vi "SIAM-DecodeDigitalReturn.vi"(10 "?":i32 format="%.0b", 11 "Array 2":T1(array[cluster])=[{"Digital-out"=enum."cam1", "Boolean"=FALSE}, {"Digital-out"=enum."cam2", "Boolean"=FALSE}, {"Digital-out"=enum."led2", "Boolean"=FALSE}, {"Digital-out"=enum."led3", "Boolean"=FALSE}, {"Digital-out"=enum."led4", "Boolean"=FALSE}, {"Digital-out"=enum."led5", "Boolean"=FALSE}, {"Digital-out"=enum."led5", "Boolean"=FALSE}, {"Digital-out"=enum."led7", "Boolean"=FALSE}, {"Digital-out"=enum."led8", "Boolean"=FALSE}, {"Digital-out"=enum."durchR", "Boolean"=FALSE}, {"Digital-out"=enum."tsm-pwr", "Boolean"=FALSE}, {"Digital-out"=enum."dc-pwr", "Boolean"=FALSE}, {"Digital-out"=enum."laser-pwr", "Boolean"=FALSE}, {"Digital-out"=enum."Laser0", "Boolean"=FALSE}, {"Digital-out"=enum."Laser1", "Boolean"=FALSE}, {"Digital-out"=enum."Laser2", "Boolean"=FALSE}, {"Digital-out"=enum."Laser3", "Boolean"=FALSE}, {"Digital-out"=enum."TrigOut", "Boolean"=FALSE}, {"Digital-out"=enum."SMB1", "Boolean"=FALSE}]) -> (3 "Array 3":T1(array[cluster])=[{"Digital-out"=enum."cam1", "Boolean"=FALSE}, {"Digital-out"=enum."cam2", "Boolean"=FALSE}, {"Digital-out"=enum."led2", "Boolean"=FALSE}, {"Digital-out"=enum."led3", "Boolean"=FALSE}, {"Digital-out"=enum."led4", "Boolean"=FALSE}, {"Digital-out"=enum."led5", "Boolean"=FALSE}, {"Digital-out"=enum."led5", "Boolean"=FALSE}, {"Digital-out"=enum."led7", "Boolean"=FALSE}, {"Digital-out"=enum."led8", "Boolean"=FALSE}, {"Digital-out"=enum."durchR", "Boolean"=FALSE}, {"Digital-out"=enum."tsm-pwr", "Boolean"=FALSE}, {"Digital-out"=enum."dc-pwr", "Boolean"=FALSE}, {"Digital-out"=enum."laser-pwr", "Boolean"=FALSE}, {"Digital-out"=enum."Laser0", "Boolean"=FALSE}, {"Digital-out"=enum."Laser1", "Boolean"=FALSE}, {"Digital-out"=enum."Laser2", "Boolean"=FALSE}, {"Digital-out"=enum."Laser3", "Boolean"=FALSE}, {"Digital-out"=enum."TrigOut", "Boolean"=FALSE}, {"Digital-out"=enum."SMB1", "Boolean"=FALSE}])   [LabVIEW 2011]
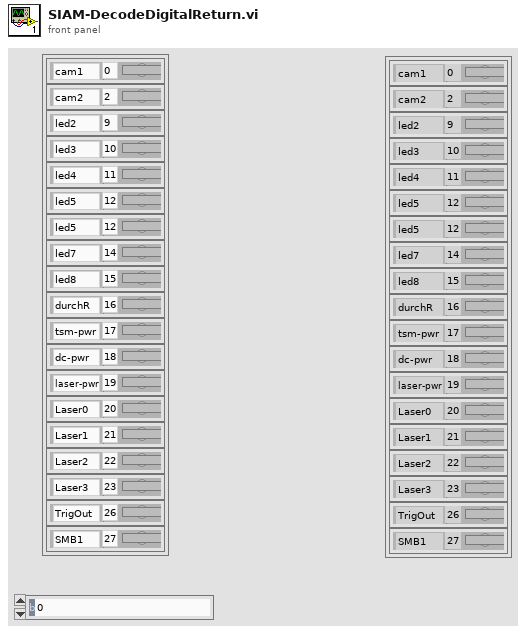
[diagram p1: front panel]
types:
  T1 = cluster{"Digital-out":enum8{"cam1", "cam1-ready?", "cam2", "cam2-ready?", "tmsx?", "tsmy?", "tsm3?", "lid?", "led1", "led2", "led3", "led4", "led5", "led6", "led7", "led8", "durchR", "tsm-pwr", "dc-pwr", "laser-pwr", "Laser0", "Laser1", "Laser2", "Laser3", "Laser4", "LaserX", "TrigOut", "SMB1", ""}, "Boolean":bool}[]
  T2 = enum8{"cam1", "cam1-ready?", "cam2", "cam2-ready?", "tmsx?", "tsmy?", "tsm3?", "lid?", "led1", "led2", "led3", "led4", "led5", "led6", "led7", "led8", "durchR", "tsm-pwr", "dc-pwr", "laser-pwr", "Laser0", "Laser1", "Laser2", "Laser3", "Laser4", "LaserX", "TrigOut", "SMB1", ""}
  T3 = cluster{"Digital-out":enum8{"cam1", "cam1-ready?", "cam2", "cam2-ready?", "tmsx?", "tsmy?", "tsm3?", "lid?", "led1", "led2", "led3", "led4", "led5", "led6", "led7", "led8", "durchR", "tsm-pwr", "dc-pwr", "laser-pwr", "Laser0", "Laser1", "Laser2", "Laser3", "Laser4", "LaserX", "TrigOut", "SMB1", ""}, "Boolean":bool}
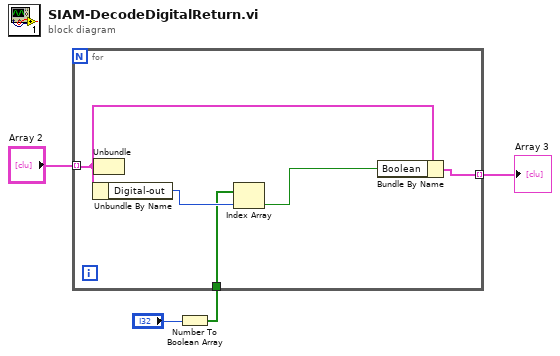
[diagram p0: block diagram]
diagram:
  n1 = Number To Boolean Array(number="?") -> (Boolean array=w1:bool[])
  n2 = for {
    tunnel: "Array 2" -> [w8] mode=indexing
    tunnel: [w9] -> w3 mode=indexing
    tunnel: w1 -> [w6]
    n3 = Unbundle By Name(w8) -> ("Digital-out"=w7:T2)
    n4 = Unbundle(w8) -> ()  [unwired: 2 out]
    n5 = Index Array(array=w6, index=w7) -> (element=w5:bool)
    n6 = Bundle By Name(cluster=w8, "Boolean"=w5) -> (w9:T3)
  }
  "Array 3" <- w3
